vi "Build Component Sub Section.vi"(4 "Dqmh Modules Overview":refnum<class "Dqmh Modules Overview.lvclass">, 5 "FrontPanelGUIOut":refnum<class "FrontPanelGUI.lvclass">, 6 "Classes Overview":refnum<class "Classes Overview.lvclass">, 7 "TAFConfiguration":refnum<class "TAFConfiguration.lvclass">[](array[class]), 8 "error in":errorcluster, 9 "Lvclass":refnum<class "Lib.lvclass">[](array[class]), 10 "Libraries":refnum<class "Lib.lvclass">[](array[class]), 11 "Dqmh Modules":refnum<class "Dqmh Module.lvclass">[](array[class])) -> (0 "error out":errorcluster, 3 "Sections":refnum<class "Section.lvclass">[](array[class]))   [LabVIEW 2021, in "TAF Proj Document Type.lvlib" / "TAF Proj.lvclass"]
uses:
  <vilib>/Wovalab/AntiDoc/Document Type/Add-ons/LabVIEW TAF Project/TAF Proj/TAF Proj.lvclass
  <vilib>/Wovalab/AntiDoc/Document Type/Add-ons/LabVIEW TAF Project/Lib/Lib.lvclass
  C:/Program Files (x86)/National Instruments/LabVIEW 2021/vi.lib/Wovalab/AntiDoc/Bloc/Bloc.lvclass
  <vilib>/Wovalab/AntiDoc/Document Type/Add-ons/LabVIEW TAF Project/Dqmh Module/Dqmh Module.lvclass
  <vilib>/Wovalab/AntiDoc/Section/Section.lvclass
  <vilib>/Wovalab/AntiDoc/Document Type/Add-ons/LabVIEW TAF Project/Classes Overview/Classes Overview.lvclass
  <vilib>/Wovalab/AntiDoc/Document Type/Add-ons/LabVIEW TAF Project/Dqmh Modules Overview/Dqmh Modules Overview.lvclass
  <vilib>/Wovalab/AntiDoc/Document Type/Add-ons/LabVIEW TAF Project/TAFConfiguration/TAFConfiguration.lvclass
  <vilib>/Wovalab/AntiDoc/Document Type/Add-ons/LabVIEW TAF Project/FrontPanelGUI/FrontPanelGUI.lvclass
  <vilib>/Wovalab/AsciiDoc for LabVIEW/Diagram/Type--enum.ctl
  <vilib>/Wovalab/AsciiDoc for LabVIEW/Admonition/Types--enum.ctl
  <vilib>/Wovalab/AsciiDoc for LabVIEW/Paragraph/Paragraph.lvclass
  C:/Program Files (x86)/National Instruments/LabVIEW 2021/vi.lib/Wovalab/AsciiDoc for LabVIEW/Adoc-Bloc/Bloc.lvclass
  <vilib>/Wovalab/AsciiDoc for LabVIEW/Diagram/Diagram.lvclass
  <vilib>/Wovalab/AsciiDoc for LabVIEW/Admonition/Admonition.lvclass
  <vilib>/Wovalab/AntiDoc/Bloc/Bloc.lvclass
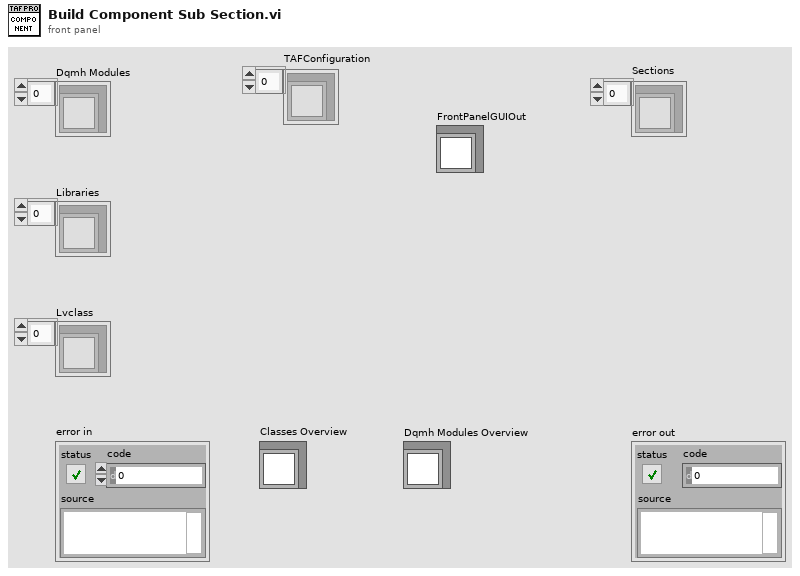
[diagram p1: front panel]
types:
  T1 = typedef "Wovalab_lib_AsciiDoctor.lvlib/Admonition.lvclass/Types--enum.ctl" = enum16{"Note", "Tip", "Important", "Warning", "Caution"}
  T2 = typedef "Wovalab_lib_AsciiDoctor.lvlib/Diagram.lvclass/Type--enum.ctl" = enum16{"a2s", "actdiag", "blockdiag", "ditaa", "erd", "graphviz", "meme", "mermaid", "msc", "nwdiag", "packetdiag", "plantuml", "rackdiag", "seqdiag", "shaape", "svgbob", "syntrax", "umlet", "vega", "vegalite", "wavedrom"}
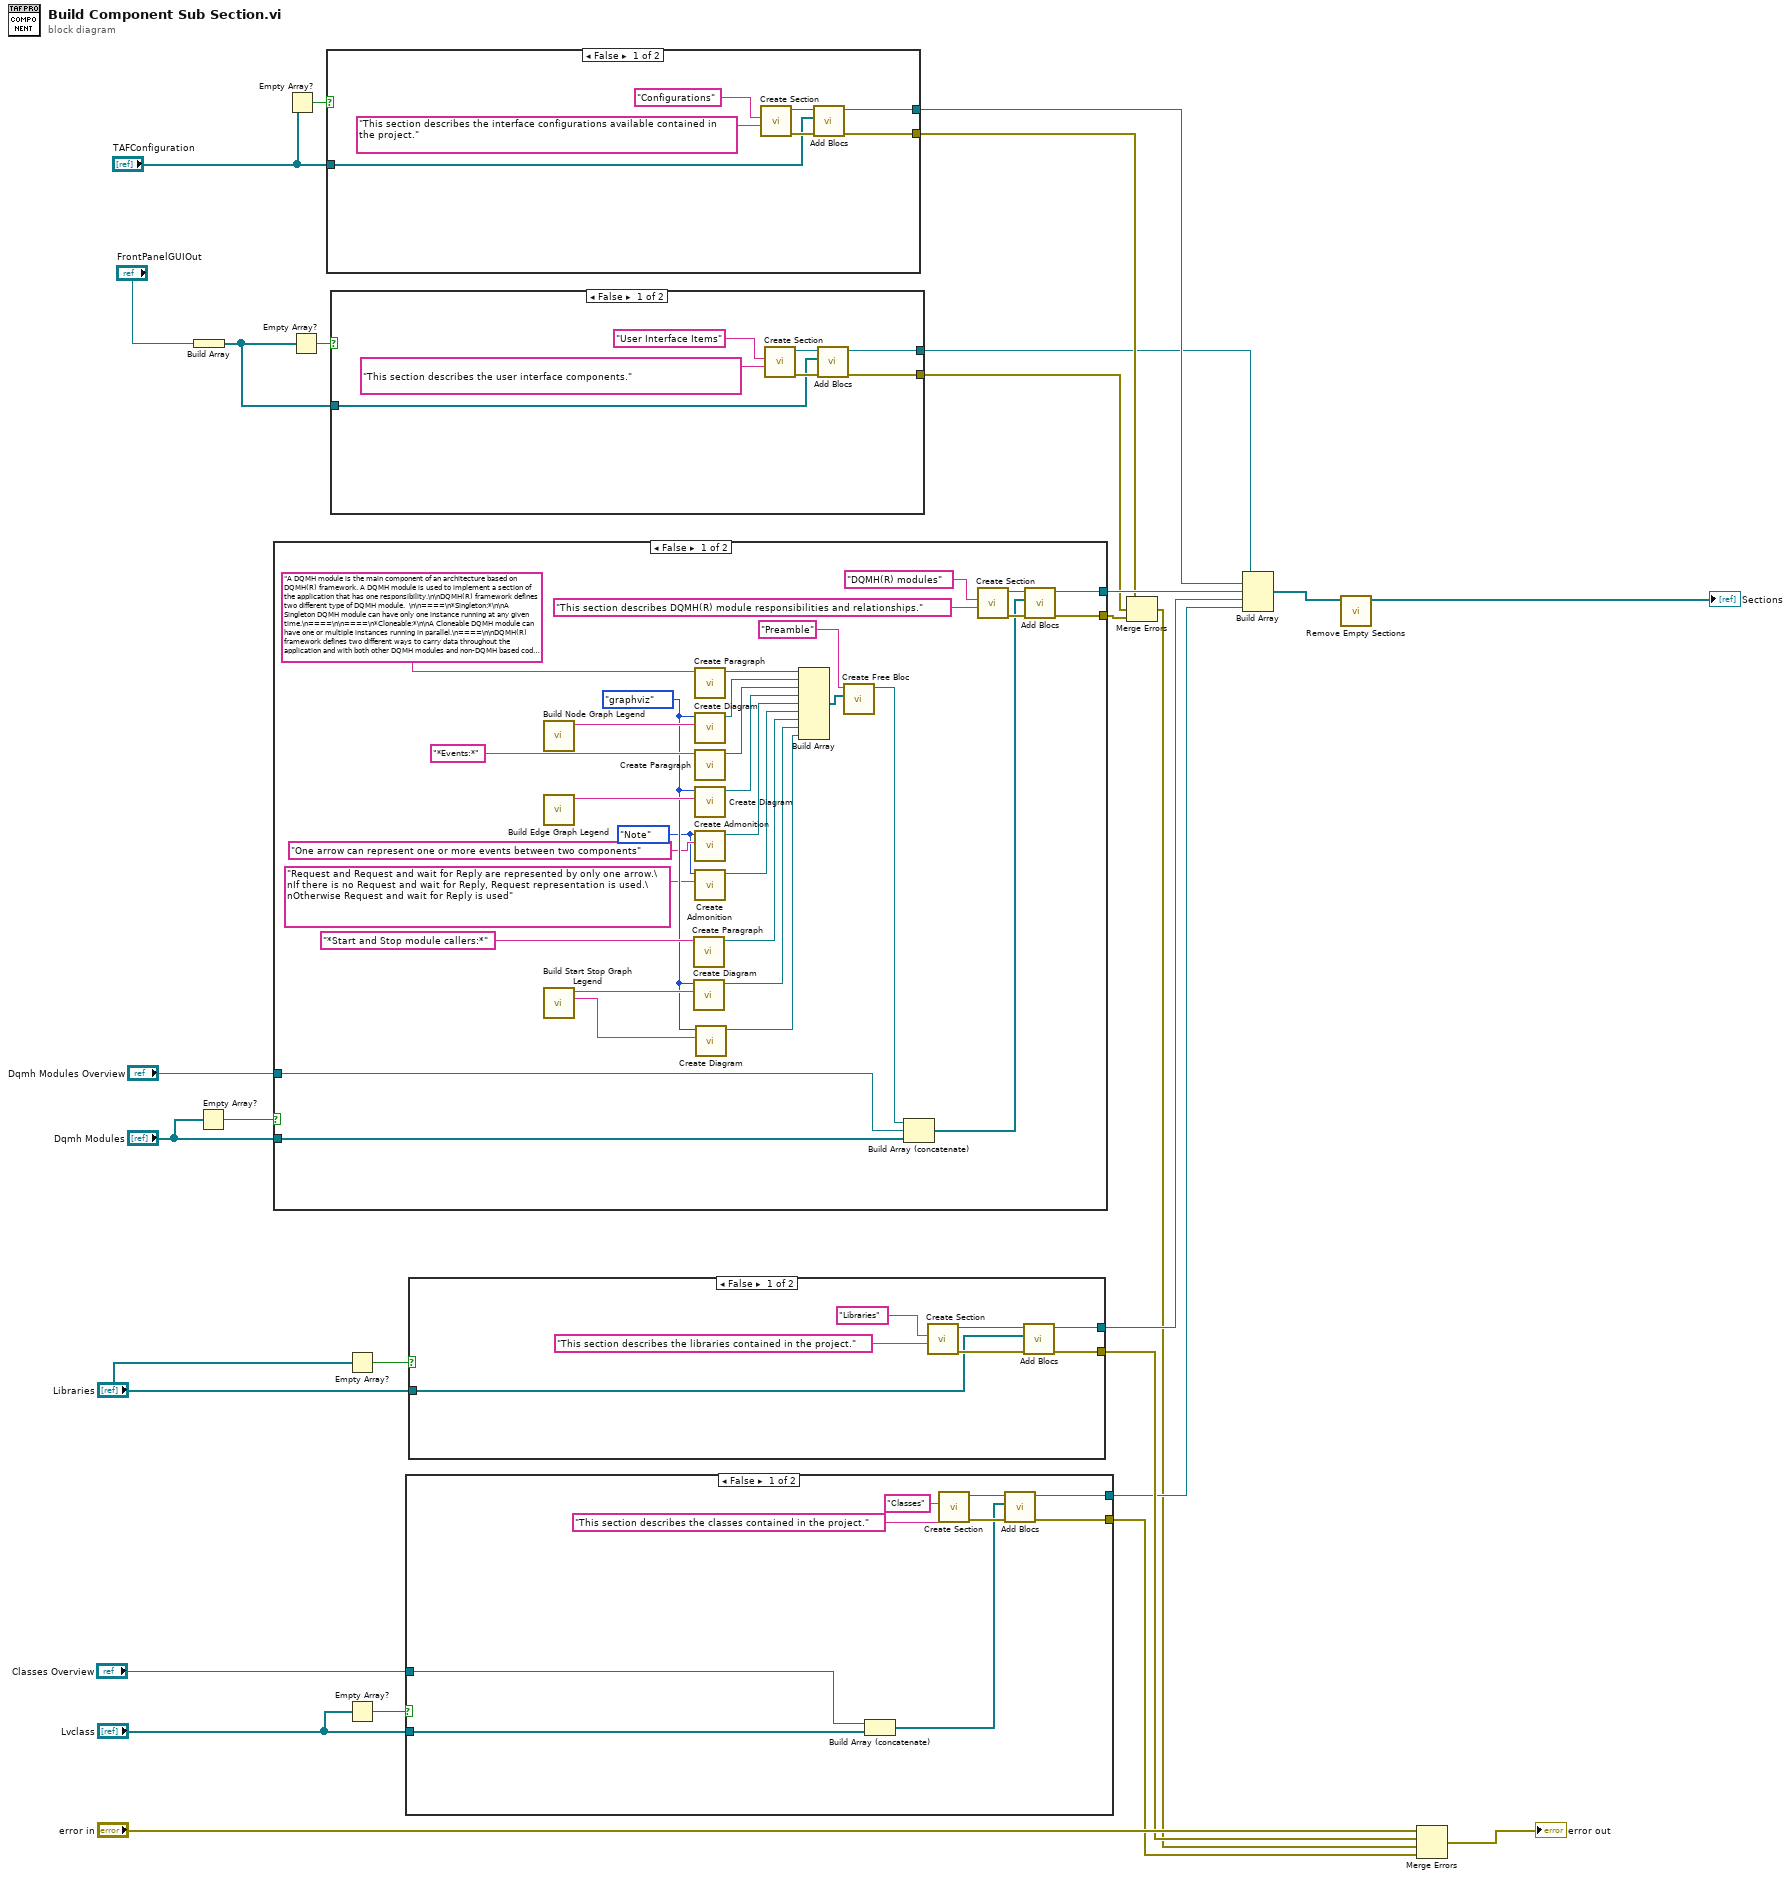
[diagram p0: block diagram]
diagram:
  n1 = Build Array("FrontPanelGUIOut") -> (w3:refnum<class "FrontPanelGUI.lvclass">[])
  n2 = Empty Array?(array="Dqmh Modules") -> (empty?=w15:bool)
  n3 = case shown="False" w15 {
    tunnel: [w59 _] -> w25
    tunnel: [w36 _] -> w22
    tunnel: "Dqmh Modules" -> [w55 _]
    tunnel: "Dqmh Modules Overview" -> [w29 _]
    frame False {
      w32 = Types--enum."Note" ("Types")
      w35 = Type--enum."graphviz" ("Diagram Type")
      n4 = call <vilib>:"Build Node Graph Legend.vi"() -> ("Node Legend Graph"=w47:string)  [unwired: 11 in]
      n5 = call <vilib>:"Build Edge Graph Legend.vi"() -> ("Edge Legend Graph"=w46:string)  [unwired: 11 in]
      n6 = call <vilib>:"Build Start Stop Graph Legend.vi"() -> ("Stop Legend Graph"=w44:string, "Start Legend Graph"=w45:string)  [unwired: 10 in]
      n7 = call <vilib>:"Create Paragraph.vi"("Content"="*Start and Stop module callers:*") -> ("Paragraph out"=w38:refnum<class "Paragraph.lvclass">)  [unwired: 9 in, 1 out]
      n8 = call <vilib>:"Create Diagram.vi"("Diagram Source Code"=w45, "Diagram Type"=w35) -> ("Diagram out"=w41:refnum<class "Diagram.lvclass">)  [unwired: 8 in, 1 out]
      n9 = call <vilib>:"Create Paragraph.vi"("Content"="A DQMH module is the main component of an architecture based on DQMH(R) framework. A DQMH module is used to implement a section of the application that has one responsibility.\n\nDQMH(R) framework defines two different type of DQMH module.  \n\n====\n*Singleton:*\n\nA Singleton DQMH module can have only one instance running at any given time.\n====\n\n====\n*Cloneable:*\n\nA Cloneable DQMH module can have one or multiple instances running in parallel.\n====\n\nDQMH(R) framework defines two different ways to carry data throughout the application and with both other DQMH modules and non-DQMH based code.\n\n====\n*Request events:*\n\nA request is a code that fires an event requesting the DQMH module to do something. Multiple locations in the code can send events to the DQMH module.\n\nRequest events are many-to-one.\n\nRequests are usually named using imperative tense.\n====\n\n====\n*Broadcast events:*\n\nA broadcast is a code that fires an event broadcasting that the DQMH module did something. Multiple Event Structures can register to handle the Broadcast Events.\n\nBroadcast Events are one-to-many.\n\nBroadcasts are usually named using past tense or passive voice.\n====\n\nNOTE: Refer to the DQMH(R) framework official http://delacor.com/documentation/dqmh-html/[documentation] to find more details on how the framework works\n\n\nThe following section gives you details on the project architecture relying on this framework.\nIt gives you an overview of the modules' interaction and detailed information on each module.\n\nGraphs used in this section have the following legend:\n\n*Components:*\n") -> ("Paragraph out"=w43:refnum<class "Paragraph.lvclass">)  [unwired: 9 in, 1 out]
      n10 = call <vilib>:"Create Diagram.vi"("Diagram Source Code"=w47, "Diagram Type"=w35) -> ("Diagram out"=w49:refnum<class "Diagram.lvclass">)  [unwired: 8 in, 1 out]
      n11 = call <vilib>:"Create Paragraph.vi"("Content"="*Events:*") -> ("Paragraph out"=w40:refnum<class "Paragraph.lvclass">)  [unwired: 9 in, 1 out]
      n12 = call <vilib>:"Create Diagram.vi"("Diagram Source Code"=w46, "Diagram Type"=w35) -> ("Diagram out"=w48:refnum<class "Diagram.lvclass">)  [unwired: 8 in, 1 out]
      n13 = call <vilib>:"Create Admonition.vi"("Content"="One arrow can represent one or more events between two components", "Types"=w32) -> ("Admonition out"=w34:refnum<class "Admonition.lvclass">)  [unwired: 8 in, 1 out]
      n14 = call <vilib>:"Create Admonition.vi"("Content"="Request and Request and wait for Reply are represented by only one arrow.\nIf there is no Request and wait for Reply, Request representation is used.\nOtherwise Request and wait for Reply is used", "Types"=w32) -> ("Admonition out"=w31:refnum<class "Admonition.lvclass">)  [unwired: 8 in, 1 out]
      n15 = call <vilib>:"Create Diagram.vi"("Diagram Source Code"=w44, "Diagram Type"=w35) -> ("Diagram out"=w42:refnum<class "Diagram.lvclass">)  [unwired: 8 in, 1 out]
      n16 = Build Array(w43, w49, w40, w48, w34, w31, w38, w41, w42) -> (w53:refnum<class "Bloc.lvclass">[])
      n17 = call <vilib>:"Create Free Bloc.vi"("Content"=w53, "Name"="Preamble") -> ("Bloc out"=w51:refnum<class "Bloc.lvclass">)  [unwired: 8 in, 1 out]
      n18 = Build Array (concatenate)(w51, w29, w55) -> (w54:refnum<class "Bloc.lvclass">[])
      n19 = call <vilib>:"Create Section.vi"("Description"="This section describes DQMH(R) module responsibilities and relationships.", "Name"="DQMH(R) modules") -> ("error out"=w60:errorcluster, "Section out"=w58:refnum<class "Section.lvclass">)  [unwired: 8 in]
      n20 = call <vilib>:"Add Blocs.vi"("error in (no error)"=w60, "Blocs"=w54, "Section in"=w58) -> ("error out"=w59:errorcluster, "Section out"=w36:refnum<class "Section.lvclass">)  [unwired: 7 in]
    }
    frame True {
    }
  }
  n21 = Empty Array?(array="TAFConfiguration") -> (empty?=w10:bool)
  n22 = Empty Array?(array=w3) -> (empty?=w5:bool)
  n23 = case shown="False" w10 {
    tunnel: "TAFConfiguration" -> [w63 _]
    tunnel: [w62 _] -> w8
    tunnel: [w61 _] -> w6
    frame False {
      n24 = call <vilib>:"Create Section.vi"("Description"="This section describes the interface configurations available contained in the project.", "Name"="Configurations") -> ("error out"=w65:errorcluster, "Section out"=w64:refnum<class "Section.lvclass">)  [unwired: 8 in]
      n25 = call <vilib>:"Add Blocs.vi"("error in (no error)"=w65, "Blocs"=w63, "Section in"=w64) -> ("error out"=w61:errorcluster, "Section out"=w62:refnum<class "Section.lvclass">)  [unwired: 7 in]
    }
    frame True {
    }
  }
  n26 = case shown="False" w5 {
    tunnel: w3 -> [w70 _]
    tunnel: [w69 _] -> w2
    tunnel: [w68 _] -> w1
    frame False {
      n27 = call <vilib>:"Create Section.vi"("Description"="This section describes the user interface components.", "Name"="User Interface Items") -> ("error out"=w72:errorcluster, "Section out"=w71:refnum<class "Section.lvclass">)  [unwired: 8 in]
      n28 = call <vilib>:"Add Blocs.vi"("error in (no error)"=w72, "Blocs"=w70, "Section in"=w71) -> ("error out"=w68:errorcluster, "Section out"=w69:refnum<class "Section.lvclass">)  [unwired: 7 in]
    }
    frame True {
    }
  }
  n29 = Empty Array?(array="Libraries") -> (empty?=w17:bool)
  n30 = Empty Array?(array="Lvclass") -> (empty?=w19:bool)
  n31 = case shown="False" w19 {
    tunnel: [w82 _] -> w24
    tunnel: [w77 _] -> w21
    tunnel: "Lvclass" -> [w78 _]
    tunnel: "Classes Overview" -> [w75 _]
    frame False {
      n32 = Build Array (concatenate)(w75, w78) -> (w76:refnum<class "Bloc.lvclass">[])
      n33 = call <vilib>:"Create Section.vi"("Description"="This section describes the classes contained in the project.", "Name"="Classes") -> ("error out"=w83:errorcluster, "Section out"=w79:refnum<class "Section.lvclass">)  [unwired: 8 in]
      n34 = call <vilib>:"Add Blocs.vi"("error in (no error)"=w83, "Blocs"=w76, "Section in"=w79) -> ("error out"=w82:errorcluster, "Section out"=w77:refnum<class "Section.lvclass">)  [unwired: 7 in]
    }
    frame True {
    }
  }
  n35 = case shown="False" w17 {
    tunnel: [w89 _] -> w26
    tunnel: [w84 _] -> w23
    tunnel: "Libraries" -> [w87 _]
    frame False {
      n36 = call <vilib>:"Create Section.vi"("Description"="This section describes the libraries contained in the project.", "Name"="Libraries") -> ("error out"=w90:errorcluster, "Section out"=w88:refnum<class "Section.lvclass">)  [unwired: 8 in]
      n37 = call <vilib>:"Add Blocs.vi"("error in (no error)"=w90, "Blocs"=w87, "Section in"=w88) -> ("error out"=w89:errorcluster, "Section out"=w84:refnum<class "Section.lvclass">)  [unwired: 7 in]
    }
    frame True {
    }
  }
  n38 = Merge Errors(w6, w1, w25) -> (w7:errorcluster)
  n39 = Build Array(w2, w8, w22, w23, w21) -> (w11:refnum<class "Section.lvclass">[])
  n40 = call <vilib>:"Remove Empty Sections .vi"("Array in"=w11) -> ("Array out"=→"Sections":refnum<class "Section.lvclass">[])  [unwired: 10 in]
  n41 = Merge Errors("error in", w26, w7, w24) -> (→"error out":errorcluster)
